vi "get_curr_position.vi"(8 "error in (no error)":errorcluster, 11 "dummyStageRapid in":refnum<class "dummyStageRapid.lvclass">) -> (0 "error out":errorcluster, 2 "readback position":dbl[](array[numeric]), 3 "dummyStageRapid out":refnum<class "dummyStageRapid.lvclass">)   [LabVIEW 2019, in "dummyStageRapid.lvlib" / "dummyStageRapid.lvclass"]
uses:
  dummyStageRapid.lvclass
panel:
  out "text":string
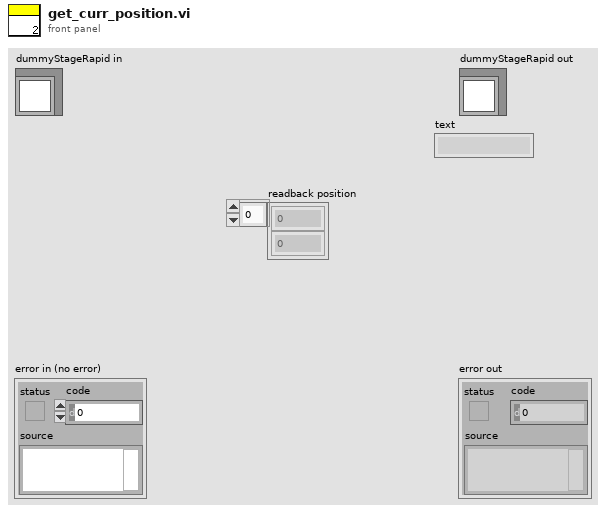
[diagram p1: front panel]
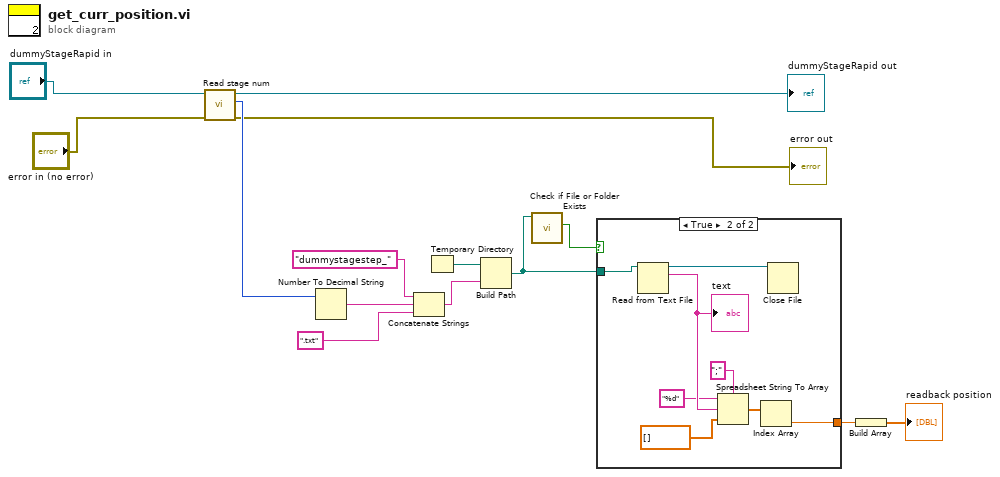
[diagram p0: block diagram]
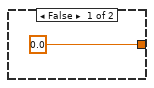
[diagram p2: hidden frame]
diagram:
  n1 = call-dynamic "Read stage num.vi"("error in (no error)"="error in (no error)", "_stage in"="dummyStageRapid in") -> ("error out"=→"error out":errorcluster, "stage num"=w8:u8, "_stage out"=→"dummyStageRapid out":refnum<class "dummyStageRapid.lvclass">)  [unwired: 7 in]
  n2 = Number To Decimal String(number=w8) -> (decimal integer string=w13:string)  [unwired: 1 in]
  n3 = Concatenate Strings("dummystagestep_", w13, ".txt") -> (w11:string)
  n4 = Temporary Directory() -> (w10:path)
  n5 = Build Path(base path=w10, name or relative path=w11) -> (appended path=w3:path)
  n6 = call <vilib>:"Check if File or Folder Exists.vi"("path"=w3) -> ("file or folder exists?"=w4:bool)  [unwired: 8 in, 2 out]
  n7 = case shown="True" w4 {
    tunnel: w3 -> [_ w22]
    tunnel: [0.0 w17] -> w2
    frame False {
    }
    frame True {
      n8 = Read from Text File(file (use dialog)=w22) -> (refnum out=w23:refnum<file>, text=w21:string)  [unwired: 3 in, 2 out]
      "text" <- w21
      n9 = Spreadsheet String To Array(delimiter (Tab)=";", format string="%d", spreadsheet string=w21, array type (2D Dbl)=dbl[] []) -> (array=w18:dbl[])
      n10 = Index Array(array=w18) -> (element=w17:dbl)  [unwired: 1 in]
      n11 = Close File(refnum=w23) -> ()  [unwired: 1 in, 2 out]
    }
  }
  n12 = Build Array(w2) -> (→"readback position":dbl[])
